vi "SweepSettings.vi"(11 "FPGA VI Reference Out":T1) -> ()   [LabVIEW 2012]
uses:
  <vilib>/rvi/interface/nirviReadWriteControl/nirviReadWriteControl.xnode
  <vilib>/DAQmx/create/channels.llb/DAQmx Create Channel (AI-Voltage-Basic).vi
  <vilib>/DAQmx/read.llb/DAQmx Read (Analog DBL 1Chan 1Samp).vi
  <vilib>/Utility/file.llb/Write To Spreadsheet File (DBL).vi
  AODRef.ctl
panel:
  in  "physical channels":tag="PXI1Slot2/ai0"
  out "Executing":bool=TRUE
  in  "Execute":bool
  in  "stop":bool
  in  "Steps":T2={"XHP"=16, "XLP"=1, "YHP"=1, "YLP"=1} {"XHP" min=1 max=50; "XLP" min=1 max=50; "YHP" min=1 max=50; "YLP" min=1 max=50}
  in  "Center Frequencies":T2={"XHP"=805306367, "XLP"=858993459, "YHP"=805306367, "YLP"=858993459} {"XHP" format="%x"; "XLP" format="%x"; "YHP" format="%x"; "YLP" format="%x"}
  in  "Delta":T2={"XHP"=100000, "XLP"=0, "YHP"=0, "YLP"=0}
  in  "Save":bool
  out "Data":dbl[](array[numeric])
  out "Array":dbl[][][][](array[numeric])
  in  "task in":refnum<k21>
  out "Bad Coordinate":bool
  in  "Pause (ms)":dbl
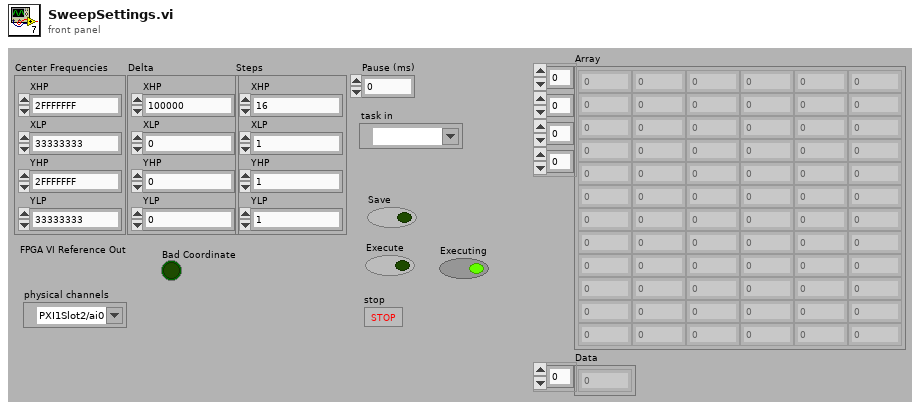
[diagram p1: front panel]
types:
  T1 = typedef "AODRef.ctl" = refnum<k20>
  T2 = cluster{"XHP":i32, "XLP":i32, "YHP":i32, "YLP":i32}
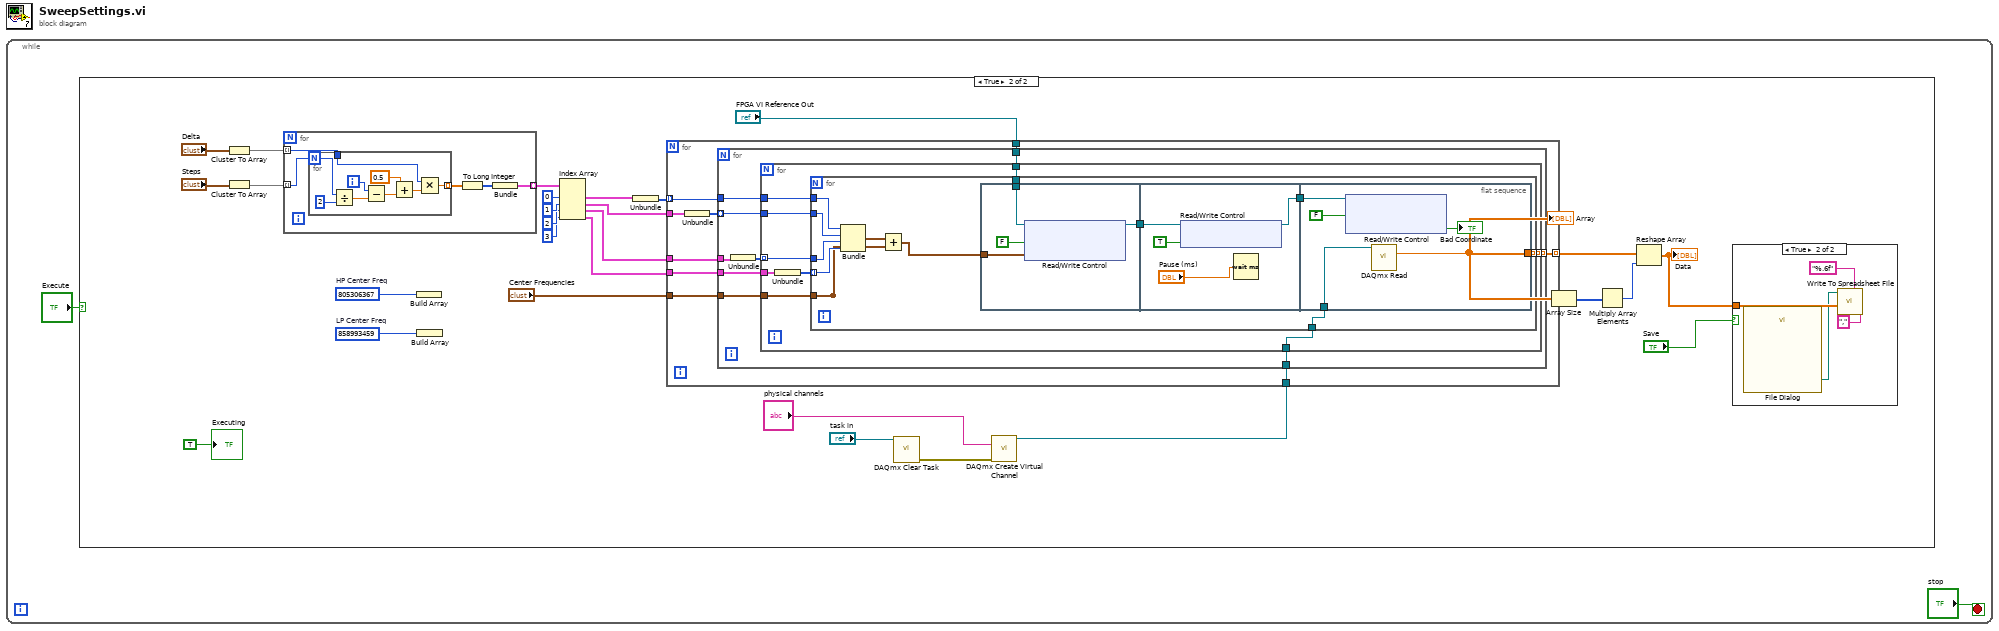
[diagram p0: block diagram]
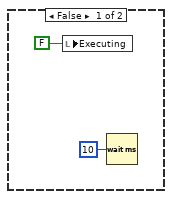
[diagram p2: hidden frame]
diagram:
  n1 = while {
    stop <- "stop" stop-if-true
    n2 = case shown="True" "Execute" {
      frame False {
        n3 = local write "Executing"(FALSE ("Executing")) -> ()
        n4 = Wait (ms)(milliseconds to wait=u32 10) -> ()  [unwired: 1 out]
      }
      frame True {
        w27 = u32 805306367  # HP Center Freq
        w26 = u32 858993459  # LP Center Freq
        n5 = Cluster To Array(cluster="Delta") -> (array=w18:i32[])
        n6 = Cluster To Array(cluster="Steps") -> (array=w20:i32[])
        n7 = for {
          tunnel: w18 -> [w36] mode=indexing
          tunnel: w20 -> [w37] mode=indexing
          tunnel: [w33] -> w10 mode=indexing
          n8 = for {
            N: w37 -> [w45]
            tunnel: w36 -> [w39]
            tunnel: [w38] -> w35 mode=indexing
            i -> [w46]
            n9 = Divide(x=w45, y=2) -> (x/y=w43:dbl)
            n10 = Subtract(x=w46, y=w43) -> (x-y=w42:dbl)
            n11 = Add(x=0.5, y=w42) -> (x+y=w40:dbl)
            n12 = Multiply(x=w39, y=w40) -> (x*y=w38:dbl)
          }
          n13 = To Long Integer(number=w35) -> (32bit integer=w34:i32[])
          n14 = Bundle(w34) -> (w33:cluster{i32[]})  [unwired: 1 in]
        }
        n15 = Build Array(w27) -> ()  [unwired: 1 out]
        n16 = Build Array(w26) -> ()  [unwired: 1 out]
        n17 = Index Array(array=w10, index #1=0 ("index (row)"), index #2=1 ("index (row)"), index #3=2 ("index (row)"), index #4=3 ("index (row)")) -> (element #1=w9:cluster{i32[]}, element #2=w13:cluster{i32[]}, element #3=w12:cluster{i32[]}, element #4=w11:cluster{i32[]})
        n18 = Unbundle(w9) -> (w8:i32[])
        n19 = call <vilib>:"DAQmx Clear Task.vi"("task in"="task in") -> ("error out"=w31:errorcluster)  [unwired: 14 in]
        n20 = call-poly <vilib>:"DAQmx Create Virtual Channel.vi"("physical channels"="physical channels", "error in"=w31) -> ("task out"=w29:refnum<k21>)  [unwired: 12 in, 1 out]
        n21 = for {
          tunnel: w13 -> [w54]
          tunnel: w12 -> [w59]
          tunnel: w29 -> [w58]
          tunnel: [w57] -> w25 mode=indexing
          tunnel: w11 -> [w56]
          tunnel: w8 -> [w55] mode=indexing
          tunnel: "FPGA VI Reference Out" -> [w52]
          tunnel: "Center Frequencies" -> [w51]
          n22 = Unbundle(w54) -> (w53:i32[])
          n23 = for {
            tunnel: w59 -> [w63]
            tunnel: w55 -> [w68]
            tunnel: w58 -> [w67]
            tunnel: [w66] -> w57 mode=indexing
            tunnel: w56 -> [w65]
            tunnel: w53 -> [w64] mode=indexing
            tunnel: w52 -> [w61]
            tunnel: w51 -> [w60]
            n24 = Unbundle(w63) -> (w62:i32[])
            n25 = for {
              tunnel: w65 -> [w72]
              tunnel: w68 -> [w77]
              tunnel: w64 -> [w76]
              tunnel: w67 -> [w75]
              tunnel: [w74] -> w66 mode=indexing
              tunnel: w62 -> [w73] mode=indexing
              tunnel: w61 -> [w70]
              tunnel: w60 -> [w69]
              n26 = Unbundle(w72) -> (w71:i32[])
              n27 = for {
                tunnel: w73 -> [w82]
                tunnel: w77 -> [w84]
                tunnel: w76 -> [w83]
                tunnel: w75 -> [w88]
                tunnel: [w87] -> w74 mode=indexing
                tunnel: w71 -> [w81] mode=indexing
                tunnel: w70 -> [w85]
                tunnel: [w79] -> _
                tunnel: w69 -> [w79]
                n28 = Bundle(w84, w83, w82, w81) -> (w80:cluster{i32, i32, i32, i32})  [unwired: 1 in]
                n29 = Add(x=w80, y=w79) -> (x+y=w78:cluster{i32, i32, i32, i32})
                n30 = flat-sequence {
                  tunnel: [w92] -> w89
                  tunnel: w85 -> [w91]
                  tunnel: w78 -> [w90]
                  tunnel: w89 -> [w96]
                  tunnel: [w94] -> w86
                  tunnel: w88 -> [w101]
                  tunnel: [w100] -> w87
                  tunnel: w86 -> [w99]
                  frame #0 {
                    n31 = xnode "Read/Write Control"("FPGA VI Reference In"=w91, "Debug.SetCoordinate"=FALSE ("SetCoordinate"), "Debug.Coordinate"=w90) -> ("FPGA VI Reference Out"=w92:T1)  [unwired: 1 in, 1 out]
                  }
                  frame #1 {
                    n32 = xnode "Read/Write Control"("FPGA VI Reference In"=w96, "Debug.SetCoordinate"=TRUE ("SetCoordinate")) -> ("FPGA VI Reference Out"=w94:T1)  [unwired: 1 in, 1 out]
                    n33 = Wait (ms)(milliseconds to wait="Pause (ms)") -> ()  [unwired: 1 out]
                  }
                  frame #2 {
                    n34 = xnode "Read/Write Control"("FPGA VI Reference In"=w99, "Debug.SetCoordinate"=FALSE ("SetCoordinate")) -> ("Error.OutOfRange"=→"Bad Coordinate":bool)  [unwired: 1 in, 2 out]
                    n35 = call-poly <vilib>:"DAQmx Read.vi"("task/channels in"=w101) -> ("data"=w100:dbl)  [unwired: 12 in, 2 out]
                  }
                }
              }
            }
          }
        }
        "Array" <- w25
        n36 = Array Size(array=w25) -> (size(s)=w28:i32[])
        n37 = Multiply Array Elements(1:w28) -> (0:w24:i32)
        n38 = Reshape Array(w25, w24) -> (w23:dbl[])
        "Data" <- w23
        n39 = case shown="True" "Save" {
          tunnel: w23 -> [_ w50]
          frame False {
          }
          frame True {
            n40 = call "File Dialog"() -> ("selected path"=w49:path)  [unwired: 12 in, 3 out]
            n41 = call-poly <vilib>:"Write To Spreadsheet File.vi"("delimiter (\\t)"="," ("delimiter (\\t)"), "format (%.3f)"="%.6f", "1D data"=w50, "file path (dialog if empty)"=w49) -> ()  [unwired: 4 in, 1 out]
          }
        }
        "Executing" <- TRUE
      }
    }
  }
